vi "16TwosCompl_To_Decimal.vi"(1 "16 bit":bool[](array[boolean])) -> (0 "Decimal by traditional way":i32)   [LabVIEW 2011]
panel:
  # "LSB"
  # "MSB"
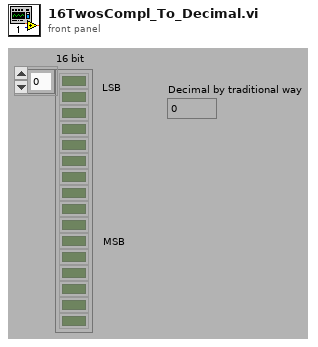
[diagram p1: front panel]
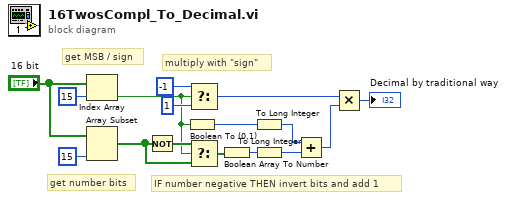
[diagram p0: block diagram]
diagram:
  # "multiply with \"sign\""
  # "IF number negative THEN invert bits and add 1"
  # "get number bits"
  # "get MSB / sign"
  n1 = Index Array(array="16 bit", index=15) -> (element=w3:bool)
  n2 = Array Subset(array="16 bit", length=15) -> (w2:bool[])  [unwired: 1 in]
  n3 = Not(x=w2) -> (.not. x?=w12:bool[])
  n4 = Boolean To (0,1)(Boolean=w3) -> (0, 1=w10:i16)
  n5 = Select(t=-1, s=w3, f=1) -> (s? t:f=w7:i32)
  n6 = Select(t=w12, s=w3, f=w2) -> (s? t:f=w1:bool[])
  n7 = Boolean Array To Number(Boolean array=w1) -> (number=w13:u32)
  n8 = To Long Integer(number=w10) -> (32bit integer=w4:i32)
  n9 = To Long Integer(number=w13) -> (32bit integer=w11:i32)
  n10 = Add(x=w4, y=w11) -> (x+y=w6:i32)
  n11 = Multiply(x=w7, y=w6) -> (x*y=→"Decimal by traditional way":i32)
